vi "TaskFor_MapGuide_Data_msg.vi"(8 "error in (no error)":errorcluster caption="错误输入（无错误）", 10 "MapGuide_Data":cluster{"X":i32, "Y":i32}, 11 "Remote Endpoint P3AT输入":refnum<class "RemoteP3AT.lvclass">) -> (0 "error out":errorcluster caption="错误输出", 3 "Remote Endpoint P3AT输出":refnum<class "RemoteP3AT.lvclass">)   [LabVIEW 2014]
uses:
  RemoteP3AT.lvclass
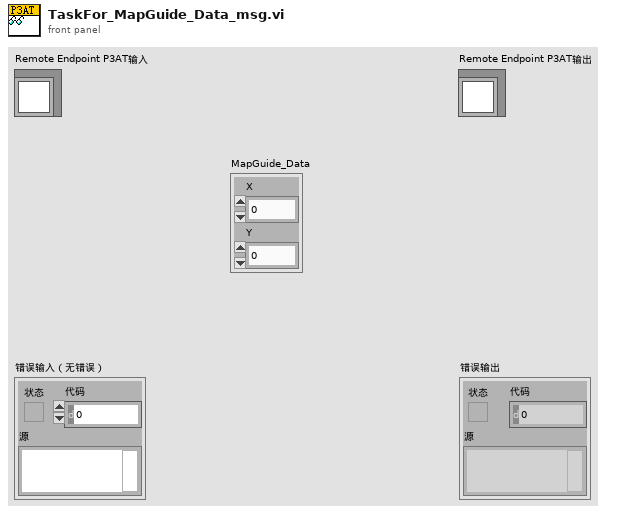
[diagram p1: front panel]
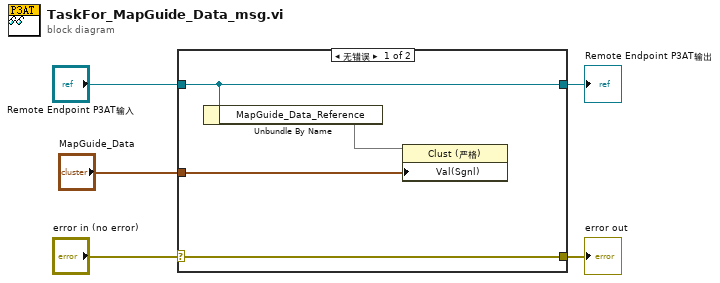
[diagram p0: block diagram]
diagram:
  n1 = case shown="无错误" "error in (no error)" {
    selector: "error in (no error)" -> [w9 w10]
    tunnel: [w9 w10] -> w4
    tunnel: [w8 w11] -> w2
    tunnel: "Remote Endpoint P3AT输入" -> [w8 w11]
    tunnel: "MapGuide_Data" -> [w6 _]
    frame No Error {
      n2 = Unbundle By Name(w8) -> ("MapGuide_Data_Reference"=w7)
      n3 = property class="Clust (严格)"(reference=w7, "Val(Sgnl)"=w6) -> ()  [unwired: 1 in, 2 out]
    }
    frame Error {
    }
  }
  "error out" <- w4
  "Remote Endpoint P3AT输出" <- w2
